vi "8channelConvert.vi"(8 "Port 0":T1, 14 "采样率":u32, 18 "总时间（单位ms）":dbl) -> (16 "单通道总采样点":dbl, 19 "appended array":u8[][](array[numeric]))   [LabVIEW 2021]
panel:
  out "Port Control 1":enum32{"Port 0", "Port 1", "Port 2", "Port 3"}(tab)
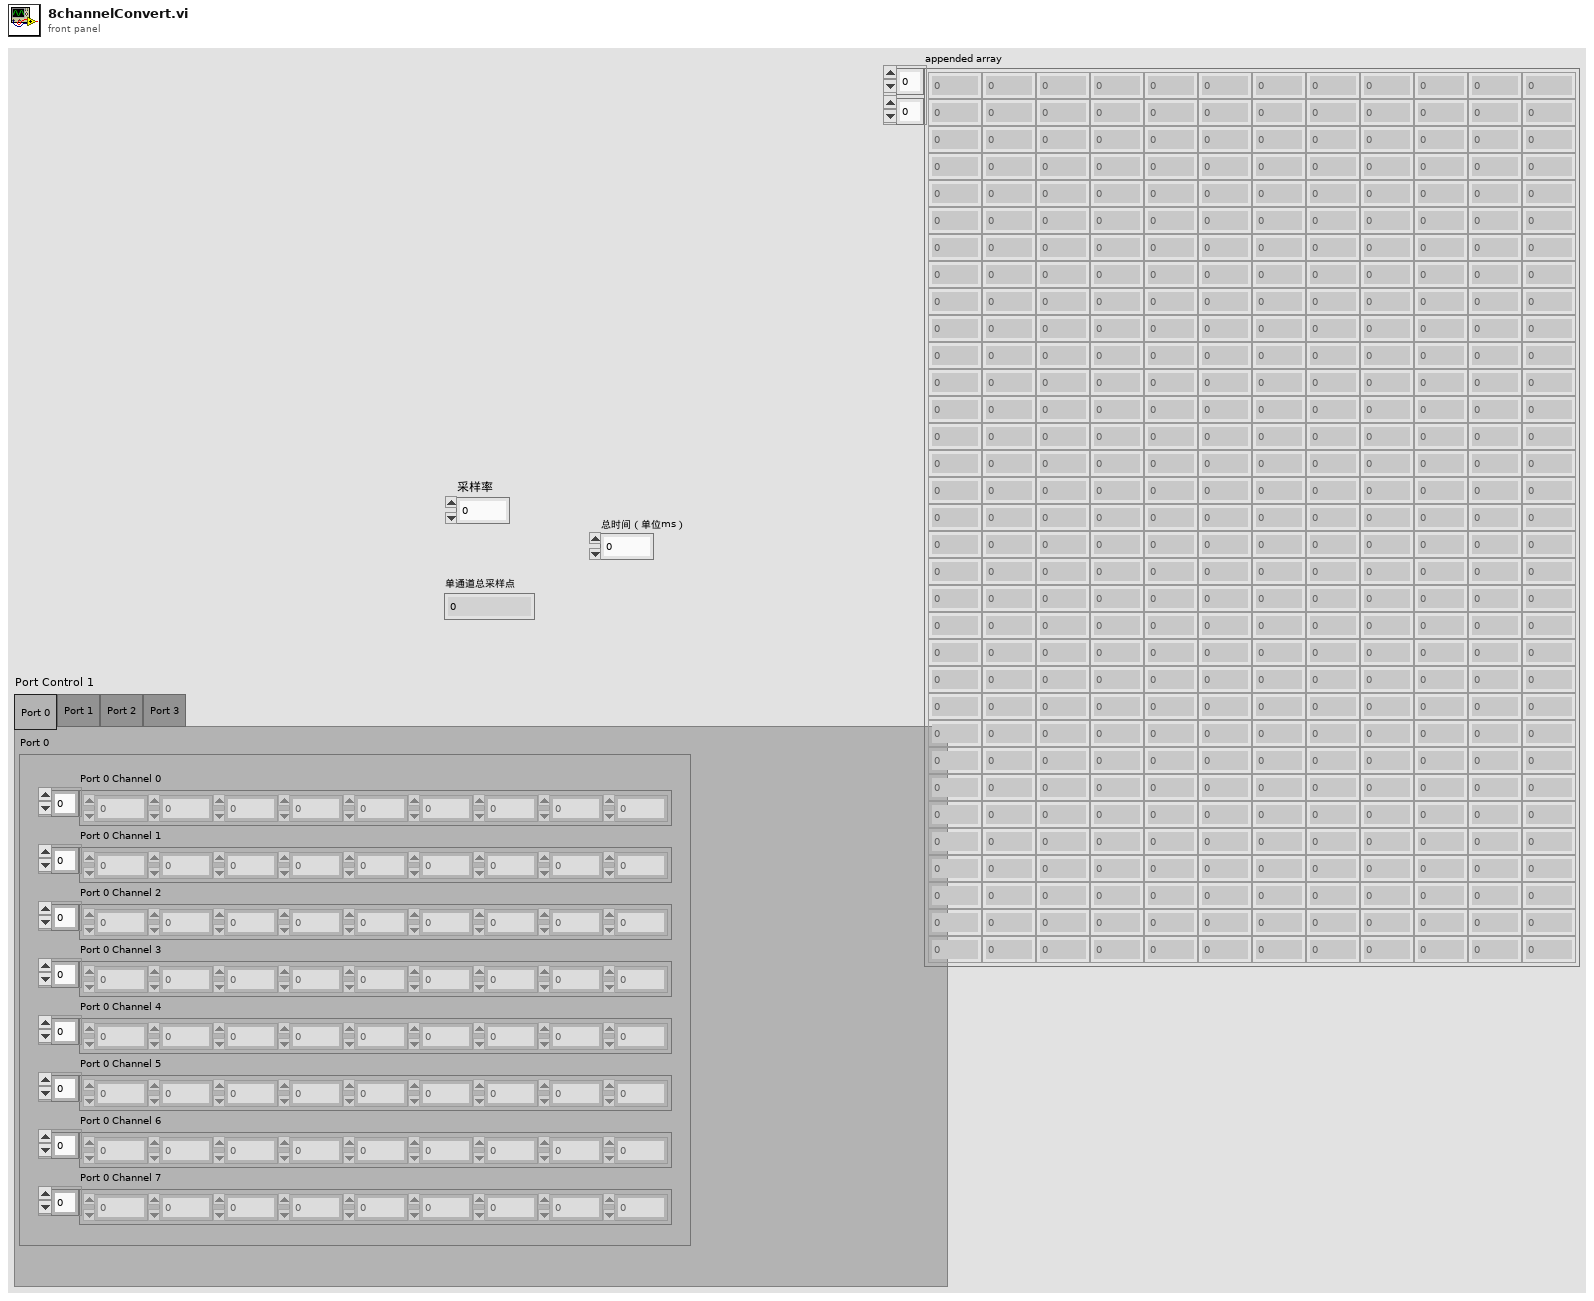
[diagram p1: front panel]
types:
  T1 = cluster{"Port 0 Channel 1":dbl[], "Port 0 Channel 2":dbl[], "Port 0 Channel 3":dbl[], "Port 0 Channel 4":dbl[], "Port 0 Channel 5":dbl[], "Port 0 Channel 6":dbl[], "Port 0 Channel 7":dbl[], "Port 0 Channel 0":dbl[]}
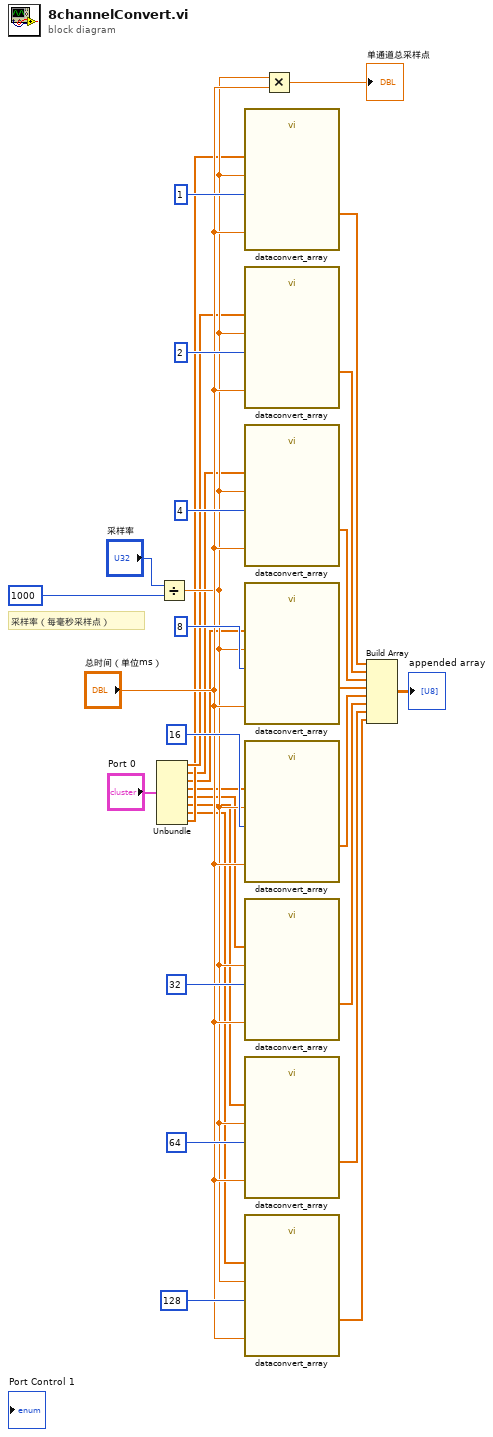
[diagram p0: block diagram]
diagram:
  # "采样率（每毫秒采样点）"
  n1 = Unbundle("Port 0") -> ("Port 0 Channel 1"=w9:dbl[], "Port 0 Channel 2"=w1:dbl[], "Port 0 Channel 3"=w7:dbl[], "Port 0 Channel 4"=w6:dbl[], "Port 0 Channel 5"=w5:dbl[], "Port 0 Channel 6"=w4:dbl[], "Port 0 Channel 7"=w3:dbl[], "Port 0 Channel 0"=w8:dbl[])
  n2 = Divide(x="采样率", y=u32 1000) -> (x/y=w11:dbl)
  n3 = call "dataconvert_array.vi"("总时间（ms）"="总时间（单位ms）", "相乘倍数"=1, "每毫秒采样点"=w11, "输入的TTL信号序列"=w8) -> ("输出编码后的TTL序列"=w29:dbl[])  [unwired: 7 in]
  n4 = call "dataconvert_array.vi"("总时间（ms）"="总时间（单位ms）", "相乘倍数"=2, "每毫秒采样点"=w11, "输入的TTL信号序列"=w9) -> ("输出编码后的TTL序列"=w25:dbl[])  [unwired: 7 in]
  n5 = call "dataconvert_array.vi"("总时间（ms）"="总时间（单位ms）", "相乘倍数"=4, "每毫秒采样点"=w11, "输入的TTL信号序列"=w1) -> ("输出编码后的TTL序列"=w23:dbl[])  [unwired: 7 in]
  n6 = call "dataconvert_array.vi"("总时间（ms）"="总时间（单位ms）", "相乘倍数"=8, "每毫秒采样点"=w11, "输入的TTL信号序列"=w7) -> ("输出编码后的TTL序列"=w22:dbl[])  [unwired: 7 in]
  n7 = call "dataconvert_array.vi"("总时间（ms）"="总时间（单位ms）", "相乘倍数"=16, "每毫秒采样点"=w11, "输入的TTL信号序列"=w6) -> ("输出编码后的TTL序列"=w20:dbl[])  [unwired: 7 in]
  n8 = call "dataconvert_array.vi"("总时间（ms）"="总时间（单位ms）", "相乘倍数"=32, "每毫秒采样点"=w11, "输入的TTL信号序列"=w5) -> ("输出编码后的TTL序列"=w18:dbl[])  [unwired: 7 in]
  n9 = call "dataconvert_array.vi"("总时间（ms）"="总时间（单位ms）", "相乘倍数"=64, "每毫秒采样点"=w11, "输入的TTL信号序列"=w4) -> ("输出编码后的TTL序列"=w16:dbl[])  [unwired: 7 in]
  n10 = call "dataconvert_array.vi"("总时间（ms）"="总时间（单位ms）", "相乘倍数"=128, "每毫秒采样点"=w11, "输入的TTL信号序列"=w3) -> ("输出编码后的TTL序列"=w14:dbl[])  [unwired: 7 in]
  n11 = Multiply(x=w11, y="总时间（单位ms）") -> (x*y=→"单通道总采样点":dbl)
  n12 = Build Array(w29, w25, w23, w22, w20, w18, w16, w14) -> (→"appended array":dbl[][])
